vi "SubVI_Broadcast_Acc_Data.vi"(8 "error in (no error)":errorcluster, 11 "Acc Data In":T1) -> (0 "error out":errorcluster)   [LabVIEW 2020]
uses:
  <extravilib>/ChannelInstances/Lossy Stream-a[.](dbl)/)Channel.ctl
  <extravilib>/ChannelInstances/Lossy Stream-a[.](dbl)/EndpointRead.vi
  Global 1.vi
  <extravilib>/ChannelInstances/Lossy Stream-a[.](dbl)/)Channel.vi
  <resource>/ChannelSupport/_ChannelSupport/WaitIfNeeded.vi
  <extravilib>/ChannelInstances/Lossy Stream-a[.](dbl).lvlib
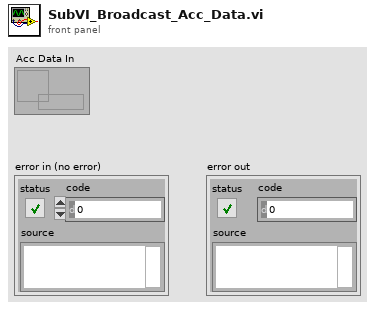
[diagram p1: front panel]
types:
  T1 = typedef "Lossy Stream-a[.](dbl).lvlib/)Channel.ctl" = refnum<queue>
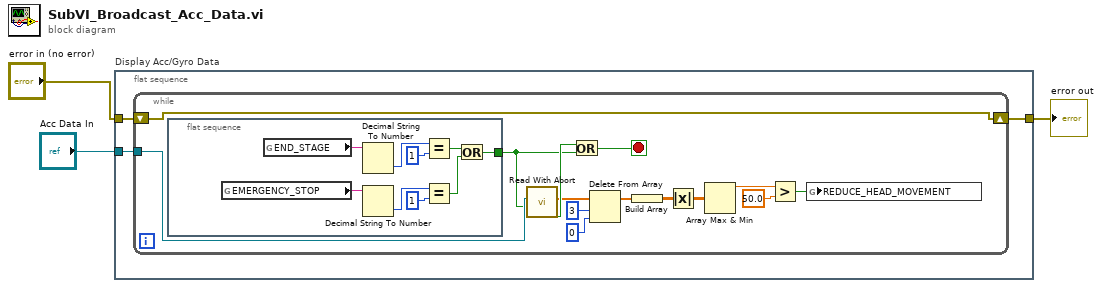
[diagram p0: block diagram]
diagram:
  n1 = flat-sequence "Display Acc/Gyro Data" {
    tunnel: [w6] -> w1
    tunnel: "error in (no error)" -> [w5]
    tunnel: "Acc Data In" -> [w4]
    frame #0 {
      n2 = while {
        shift-right: [w20] -> w6
        shift-left: w5 -> [w20]
        tunnel: w4 -> [w15]
        stop <- w19 stop-if-true
        n3 = flat-sequence {
          tunnel: [w21] -> w12
          frame #0 {
            n4 = global read "Global 1.vi" "EMERGENCY_STOP"() -> (w24:string)
            n5 = global read "Global 1.vi" "END_STAGE"() -> (w29:string)
            n6 = Decimal String To Number(string=w29) -> (number=w28:i32)  [unwired: 2 in, 1 out]
            n7 = Decimal String To Number(string=w24) -> (number=w26:i32)  [unwired: 2 in, 1 out]
            n8 = Equal?(x=w28, y=1) -> (x = y?=w22:bool)
            n9 = Equal?(x=w26, y=1) -> (x = y?=w23:bool)
            n10 = Or(x=w22, y=w23) -> (x .or. y?=w21:bool)
          }
        }
        n11 = call <extravilib>:"Read With Abort.vi"("abort"=w12, "channel"=w15) -> ("element"=w13:dbl[], "aborted?"=w14:bool)  [unwired: 3 in, 5 out]
        n12 = Or(x=w14, y=w12) -> (x .or. y?=w19:bool)
        n13 = Delete From Array(array=w13, length=3, index=0) -> (array with subset deleted=w18:dbl[])  [unwired: 1 out]
        n14 = Build Array(w18) -> (w11:dbl[][])
        n15 = Absolute Value(x=w11) -> (abs(x)=w10:dbl[][])
        n16 = Array Max & Min(array=w10) -> (max value=w9:dbl)  [unwired: 3 out]
        n17 = Greater?(x=w9, y=50.0) -> (0:w7:bool)
        n18 = global write "Global 1.vi" "REDUCE_HEAD_MOVEMENT"(w7) -> ()
      }
    }
  }
  "error out" <- w1
